vi "Stop.vi"(8 "error in (no error)":errorcluster, 11 "KUKA youBot Wheel Motor in":refnum<class "NI_Robotics_KUKA youBot Wheel Motor_EtherCAT.lvclass">) -> (0 "error out":errorcluster, 3 "KUKA youBot Wheel Motor out":refnum<class "NI_Robotics_KUKA youBot Wheel Motor_EtherCAT.lvclass">)   [LabVIEW 2017, in "NI_Robotics_KUKA youBot Host.lvlib" / "NI_Robotics_KUKA youBot Wheel Motor_EtherCAT.lvclass"]
uses:
  <vilib>/robotics/KUKA youBot/Motor/Wheel Motor EtherCAT/NI_Robotics_KUKA youBot Wheel Motor_EtherCAT.lvclass
  <vilib>/robotics/KUKA youBot/Motor/Wheel Motor EtherCAT/NI_Robotics_KUKA youBot Wheel Motor_EtherCAT.lvclass/NI_Robotics_KUKA youBot Wheel Motor_EtherCAT.ctl
  <vilib>/robotics/KUKA youBot/EtherCAT/Control Mode.ctl
  <vilib>/robotics/KUKA youBot/NI_Robotics_KUKA youBot Host.lvlib
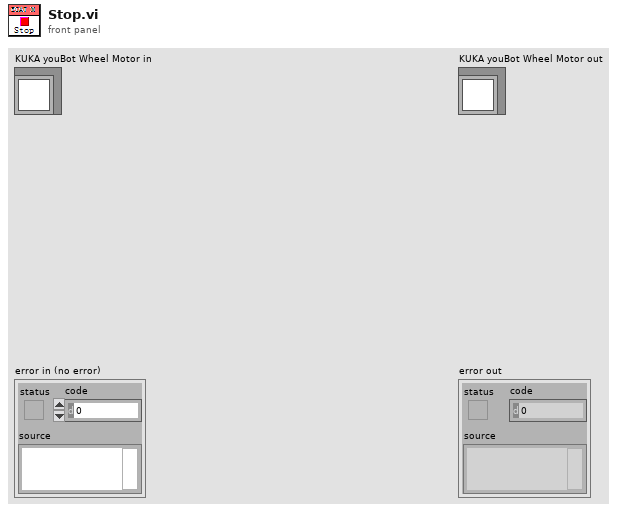
[diagram p1: front panel]
types:
  T1 = typedef "NI_Robotics_KUKA youBot Host.lvlib/Control Mode.ctl" = u8
  T2 = typedef "NI_Robotics_KUKA youBot Host.lvlib/Motor Slave Info.ctl" = cluster{"controller mode var":refnum<k21>, "reference var":refnum<k21>, "current var":refnum<k21>, "velocity var":refnum<k21>, "position var":refnum<k21>, "status var":refnum<k21>, "valid":bool, "status var type":enum16{"Int16", "Int32"}, "nodeAddr":u16, "masterHdl":T3}
  T3 = typedef "NI_Robotics_KUKA youBot Host.lvlib/Mater Handler.ctl" = i32
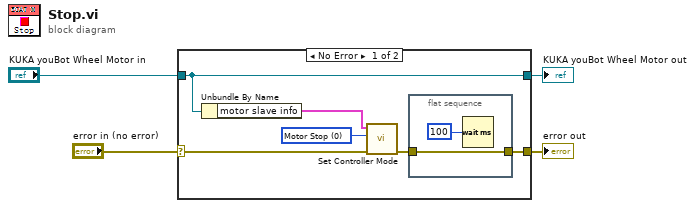
[diagram p0: block diagram]
diagram:
  n1 = case shown="No Error" "error in (no error)" {
    selector: "error in (no error)" -> [w8 w13]
    tunnel: "KUKA youBot Wheel Motor in" -> [w7 w14]
    tunnel: [w7 w14] -> w2
    tunnel: [w5 w13] -> w1
    frame No Error {
      w9 = T1 0 items=["Motor Stop", "Positioning-Mode", "Velocity-Mode", "no more action", "set position to reference", "PWM-Mode", "Current-Mode", "Initialize"] ("controller mode")
      n2 = Unbundle By Name(w7) -> ("motor slave info"=w10:T2)
      n3 = call <vilib>:"Set Controller Mode.vi"("error in (no error)"=w8, "controller mode"=w9, "motor slave info in"=w10) -> ("error out"=w6:errorcluster)  [unwired: 6 in, 2 out]
      n4 = flat-sequence {
        tunnel: [w11] -> w5
        tunnel: w6 -> [w11]
        frame #0 {
          n5 = Wait (ms)(milliseconds to wait=u32 100) -> ()  [unwired: 1 out]
        }
      }
    }
    frame Error {
    }
  }
  "KUKA youBot Wheel Motor out" <- w2
  "error out" <- w1
